vi "Query DA output source.vi"(8 "error in (no error)":errorcluster, 11 "VISA resource name":refnum<visa-resource-name>) -> (0 "error out":errorcluster, 2 "output":T1, 3 "VISA resource name out":refnum<visa-resource-name>)   [LabVIEW 2015, in "SR400.lvlib"]
doc: "AS { j }\nThe AS command reads and sets the front panel\nD/A output source. If j is absent, the D/A source is\nreturned. The parameter j may only be included if\nthe counting mode is A,B FOR T PRESET. In this\ncase, j=0 or 1 selects A or B. In all other modes,\nthe D/A output follows the count display. The\nsource may be read in all modes.\nj Output source\n0 A\n1 B\n2 A-B\n3 A+B"
uses:
  SR400.lvlib
  Typedefs/Output Source.ctl
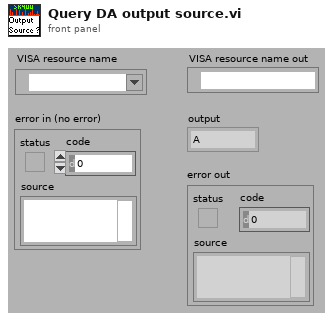
[diagram p1: front panel]
types:
  T1 = typedef "SR400.lvlib/Output Source.ctl" = enum16{"A", "B", "A - B", "A + B"}
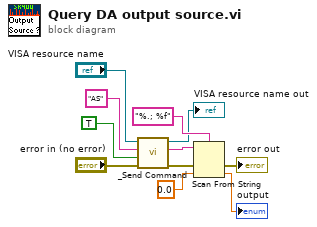
[diagram p0: block diagram]
diagram:
  n1 = call "_Send Command.vi"("error in (no error)"="error in (no error)", "Query? (F)"=TRUE, "Command"="AS" ("command"), "VISA resource name"="VISA resource name") -> ("error out"=w2:errorcluster, "Response"=w3:string, "VISA resource name out"=→"VISA resource name out":refnum<visa-resource-name>)  [unwired: 5 out]
  n2 = Scan From String(format string="%.; %f", input string=w3, error in=w2, default 1=0.0 ("default value 1")) -> (error out=→"error out":errorcluster, output 1=→"output":dbl)  [unwired: 1 in, 2 out]
